vi "faultView.vi"(10 "UserEvents in":refnum<class "UserEvents.lvclass">) -> ()   [LabVIEW 2015, in "M1M3SSSTViews.lvlib"]
uses:
  M1M3SSSTViews.lvlib
  UserEvents/UserEvents.lvclass
  UserEvents/UserEvents.lvclass/UserEvents.ctl
  Typedefs/StateSelector.ctl
  <vilib>/Utility/error.llb/DialogType.ctl
  Typedefs/M1M3SSSTypedefs.lvlib
panel:
  out "Fault":string
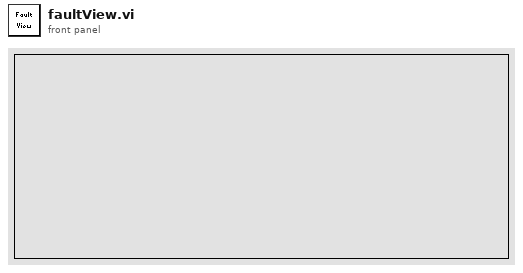
[diagram p1: front panel]
types:
  T1 = typedef "M1M3SSSTypedefs.lvlib/PubDataEvents.ctl" = cluster{"State":refnum<user-event>, "ErrorCode":refnum<user-event>, "OutputData":refnum<user-event>, "InputData":refnum<user-event>, "ControllerData":refnum<user-event>, "TestStatus":refnum<user-event>, "LogPath":refnum<user-event>, "StiffnessDataAssembly":refnum<user-event>, "PreconditioningCycle":refnum<user-event>}
  T2 = cluster{"Event Registration Refnum":refnum<event-registration>, "Event Registration Refnum":refnum<event-registration>}
  T3 = typedef "M1M3SSSTypedefs.lvlib/StateSelector.ctl" = enum16{"FaultState", "OffState", "RampingUpPressurePState", "RampingUpPressureSTState", "StandbyState", "StoppedState", "WaitingForSettledPState", "WaitingForSettledSTState"}
  T4 = typedef "DialogType.ctl" = u16
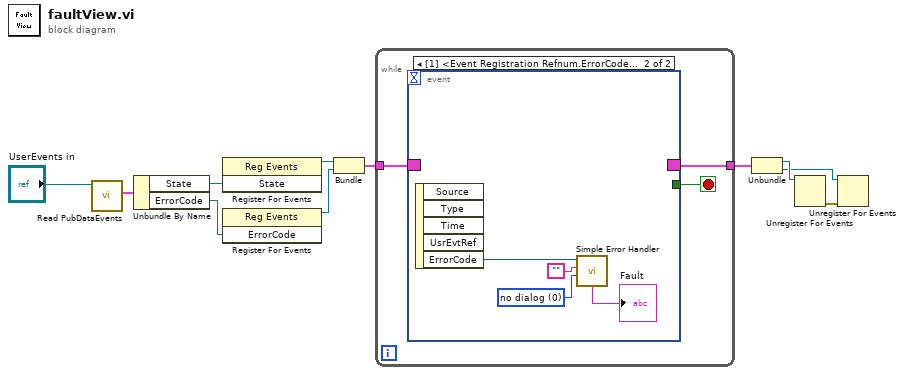
[diagram p0: block diagram]
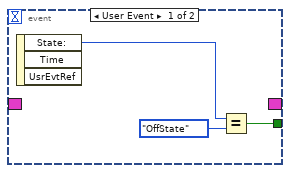
[diagram p2: hidden frame]
diagram:
  n1 = call "Read PubDataEvents.vi"("UserEvents in"="UserEvents in") -> ("PubDataEvents"=w9:T1)  [unwired: 9 in, 1 out]
  n2 = Unbundle By Name(w9) -> ("State"=w10:refnum<user-event>, "ErrorCode"=w4:refnum<user-event>)
  n3 = register-events(w10) -> (reference out=w11:refnum<event-registration>)  [unwired: 2 in, 1 out]
  n4 = register-events(w4) -> (reference out=w3:refnum<event-registration>)  [unwired: 2 in, 1 out]
  n5 = Bundle("Event Registration Refnum"=w11, "Event Registration Refnum"=w3) -> (w8:T2)  [unwired: 1 in]
  n6 = while {
    tunnel: w8 -> [w14]
    tunnel: [w13] -> w7
    stop <- w12 stop-if-true
    n7 = event shown="[1] <Event Registration Refnum.ErrorCode>: User Event" {
      selector: w14 -> [_ _]
      dyn-events: [_ _] -> w13
      timeout: _ -> [_ _]
      tunnel: [w16 _] -> w12
      event User Event {
        n8 = event-data() -> ("State:"=w15:T3)  [unwired: 1 in, 2 out]
        n9 = Equal?(x=w15, y=StateSelector."OffState") -> (x = y?=w16:bool)
      }
      event User Event {
        w21 = T4 0 items=["no dialog", "OK message", "continue or stop message", "OK message + warnings", "continue/stop + warnings"] ("type of dialog (OK msg:1)")
        n10 = event-data() -> ("ErrorCode"=w19:i32)  [unwired: 1 in, 4 out]
        n11 = call <vilib>:"Simple Error Handler.vi"("error code (no error:0)"=w19, "error source (\" \")"="", "type of dialog (OK msg:1)"=w21) -> ("message"=→"Fault":string)  [unwired: 2 in, 4 out]
      }
    }
  }
  n12 = Unbundle(w7) -> ("Event Registration Refnum"=w6:refnum<event-registration>, "Event Registration Refnum"=w2:refnum<event-registration>)
  n13 = Unregister For Events(event registration refnum=w6) -> (error out=w1:errorcluster)  [unwired: 1 in]
  n14 = Unregister For Events(event registration refnum=w2, error in=w1) -> ()  [unwired: 1 out]
